vi "Set Property.vi"(0 "video in":refnum<class "MSC Video.lvclass">, 1 "Camera Stream Property":T1=3 items=["Position msec", "Position frames", "Position avi ratio", "Frame Width", "Frame Height", "FPS", "FourCC codec", "Frame Count", "Format", "Mode", "Brightness", "Contrast", "Saturation", "Hue", "Gain", "Exposure", "Convert RGB", "White Balance U", "Rectification", "Monochrome", "Sharpness", "Auto Exposure", "Gamma", "Temperature", "Trigger", "Trigger Delay", "White Balance V", "Zoom", "Focus", "Guid", "ISO Speed", "Max DV1394", "Backlight", "Pan", "Tilt", "Rolls", "Iris", "Settings", "Buffersize"], 2 "propertyValue":dbl=1.0, 5 "error in (no error)":errorcluster) -> (14 "video out":refnum<class "MSC Video.lvclass">, 15 "propertyValue out":dbl, 19 "error out":errorcluster)   [LabVIEW 2014, in "MSC Video.lvclass"]
doc: "Sets a selected camera stream property. \nIf the value cant be set correctly, it is tried to coerce it to the nearest possible value."
uses:
  MSC Video.lvclass
  controls/Stream Property.ctl
  MSC Video.lvclass/MSC Video.ctl
  Dependencies/x86/MSC I Process32.dll
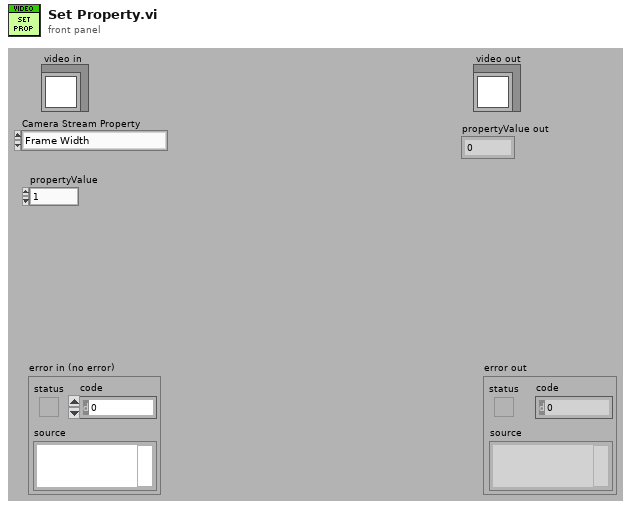
[diagram p1: front panel]
types:
  T1 = typedef "MSC Video.lvclass/Stream Property.ctl" = u16
  T2 = typedef "MSC Video.lvclass/Video.ctl" = cluster{"Pointer":u64, "CamID":i32, "File Path":path, "Network Address":string, "opened":bool}
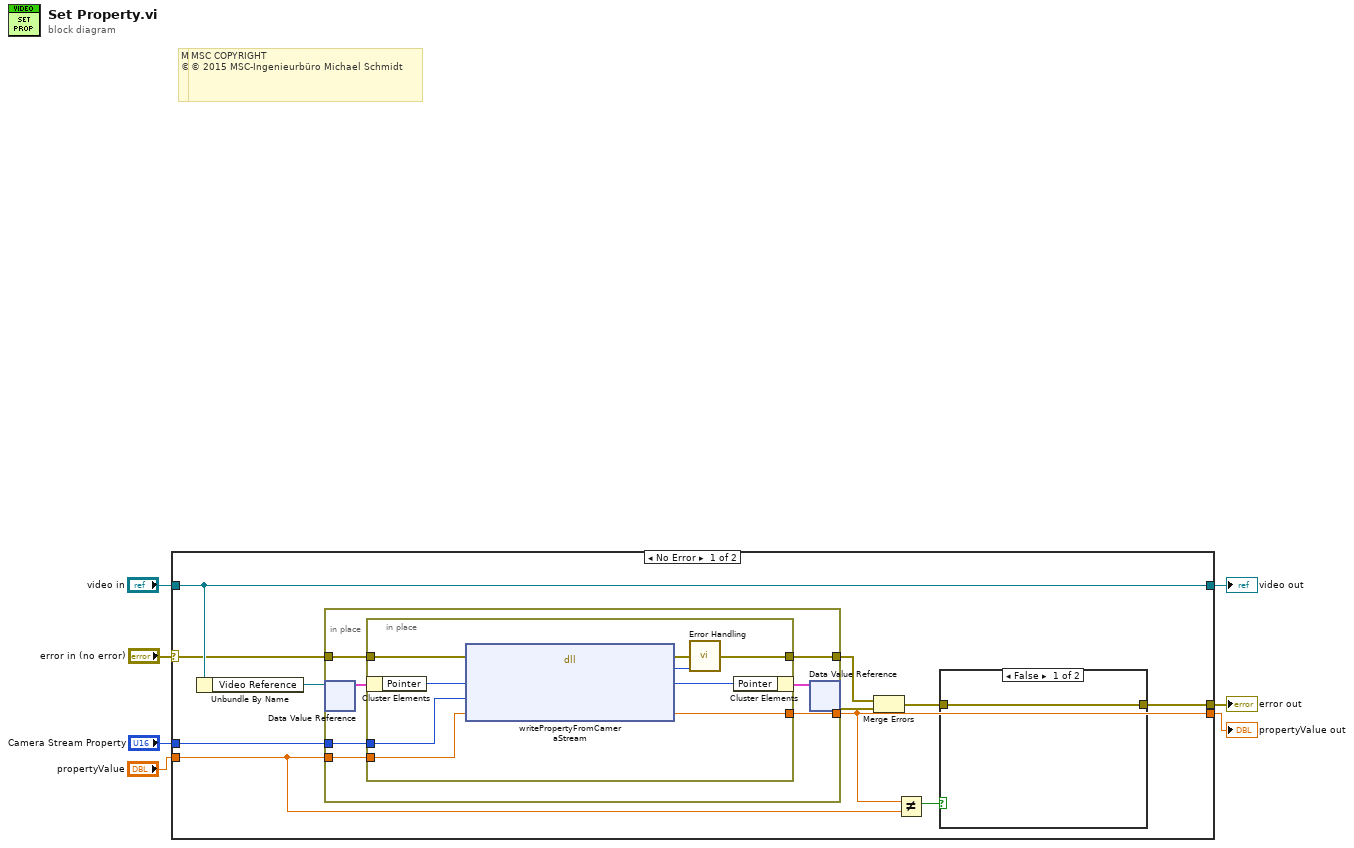
[diagram p0: block diagram]
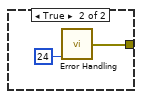
[diagram p2: hidden frame]
diagram:
  # "MSC COPYRIGHT\n© 2016 MSC-Ingenieurbüro Michael Schmidt"
  # "MSC COPYRIGHT\n© 2016 MSC-Ingenieurbüro Michael Schmidt"
  # "MSC COPYRIGHT\n© 2015 MSC-Ingenieurbüro Michael Schmidt"
  n1 = case shown="No Error" "error in (no error)" {
    selector: "error in (no error)" -> [w13 w40]
    tunnel: [w9 w40] -> w6
    tunnel: [w18 w39] -> w4
    tunnel: "video in" -> [w18 w39]
    tunnel: "Camera Stream Property" -> [w14 _]
    tunnel: "propertyValue" -> [w11 w38]
    tunnel: [w8 w38] -> w1
    frame No Error {
      n2 = Unbundle By Name(w18) -> ("Video Reference"=w15:refnum<data-value>)
      n3 = in-place {
        in-place-border: w13 -> [w26]
        in-place-border: [w25] -> w16
        in-place-border: [w24] -> w8
        in-place-border: w14 -> [w23]
        in-place-border: w11 -> [w22]
        n4 = in-place-dvr #1(w15) -> (w27:T2)  [unwired: 1 out]
        n5 = in-place {
          in-place-border: w26 -> [w31]
          in-place-border: [w37] -> w25
          in-place-border: [w33] -> w24
          in-place-border: w23 -> [w32]
          in-place-border: w22 -> [w29]
          n6 = in-place-cluster #2(w27) -> ("Pointer"=w36:u64)
          n7 = dll-call lib="C:/Users/MSC/LabVIEW Projekte/LV 2014/MSC I-Process/user.lib/MSC-I Process/Dependencies/x86/MSC I Process*.dll" fn="writePropertyFromCameraStream"(error in=w31, "streamPointer"=w36, "propertyID"=w32, "propertyValue"=w29) -> (error out=w35:errorcluster, "error"=w34:i32, "streamPointer"=w30:u64, "propertyValue"=w33:dbl)  [unwired: 3 in, 1 out]
          n8 = call "Error Handling.vi"("error in (no error)"=w35, "return type"=w34) -> ("error out"=w37:errorcluster)  [unwired: 12 in, 1 out]
          n9 = in-place-cluster #2("Pointer"=w30) -> (w28:T2)
        }
        n10 = in-place-dvr #1(w28) -> (w17:errorcluster)  [unwired: 1 out]
      }
      n11 = Merge Errors(w16, w17) -> (w10:errorcluster)
      n12 = Not Equal?(x=w8, y=w11) -> (x != y?=w12:bool)
      n13 = case shown="False" w12 {
        tunnel: w10 -> [w19 _]
        tunnel: [w19 w20] -> w9
        frame False {
        }
        frame True {
          n14 = call "Error Handling.vi"("return type"=24) -> ("error out"=w20:errorcluster)  [unwired: 13 in, 1 out]
        }
      }
    }
    frame Error {
    }
  }
  "error out" <- w6
  "video out" <- w4
  "propertyValue out" <- w1
